vi "HEWH RLT PRAT.vi"() -> ()   [LabVIEW 2023] (continued)
                n1268 = local read "Station B Test Sequence"() -> (w3112:T15[])
                n1269 = local read "Scan Rate (Seconds)"() -> (w3095:T11)
                n1270 = property on="Start/Pause test" class="Bool (strict)"("DisabledEnum"=T87."Enabled" ("Disabled")) -> ()  [unwired: 2 in, 2 out]
                n1271 = Bundle By Name(cluster=T89 {"Test Fixture Hardware"={"Power "={"Yokogawa"={"WT210"={"Sample Rate (1: 0.25s)"=0, "A Range (12: 20A)"=0, "V Range (6: 600V)"=0, "Power VISA Yokogawa WT210"=""}, "WT500"={"Power VISA Yokogawa WT500"="", "V Range (8: 1000V)"=0, "I Range (7: 40A)"=0, "Update Rate (3: 500ms)"=0}, "WT310_2"={"Sample Rate (1: 0.25s)"=0, "A Range (12: 20A)"=0, "V Range (6: 600V)"=0, "Power VISA Yokogawa WT310_2"=""}, "WT310_3"={"Sample Rate (1: 0.25s)"=0, "A Range (12: 20A)"=0, "V Range (6: 600V)"=0, "Power VISA Yokogawa WT310_3"=""}}, "Aplus"={"Aplus IP Address"="", "Remote Port"=0, "Instrument"="", "Instr Driver Revision"=""}, "Power Limits"={"Crest Factor"={"Upper Limit"=0.0, "Lower Limit"=0.0}, "Harmonic Content"={"Uthd"=0.0}, "Voltage"={"% Error"=0.0}, "Stability"={"<1 Watt "={"Wattage"=0.0, "Slope (mW/H)"=0.0}, ">1 Watt"={"1%Power/Hour"=0.0}}}, "Nominal Voltage"=0, "Time Limit (s)"=0.0, "Power Variation Limit (%)"=0.0, "Power Supply"={"Chroma 61605"="", "Use Chroma?"=FALSE}}, "Weight Scale"={"Com Options"={"IND560Scale VISA"="", "IP Address"="", "Remote Port"=0, "Setra Scale VISA"="", "GSE 350"=""}, "Select Scale"=""}, "Flow Rates"={"Laurel Cold IP Address"="", "Laurel Hot IP Address"="", "Hot Water Laurel VISA"="", "Cold Water Laurel VISA"="", "Remote Port"=0, "Laurel Communication Type"="", "Meters To Collect (Hot Cold)"="", "HOT Laurel Reference"=refnum, "COLD Laurel Reference"=refnum, "Modbus Hot Ref"=refnum}, "Analog Data"={"Agilent"={"Agilent 34972_1"="", "Agilent 34972_2"="", "Agilent 34972_3"="", "Agilent 34972_4"="", "Agilent 34972_5"="", "Agilent 34972_6"="", "Agilent Gain"=0.0, "TC Type (K,J,T)"="", "Instrument IDN?"="", "TC Channels-List"="", "Analog Channels-List"="", "Agilent Cluster Array"=[], "TC Channels-List 2"="", "Analog Channels-List 2"=""}, "Yokogawa"={"MW100"="", "Intellifaucet"=FALSE}, "Select Analog"="", "TC Coefficients"={"TC Coefficients 1"=[], "TC Coefficients 2"=[], "TC Coefficients 3"=[], "TC Coefficients 4"=[], "TC Coefficients 5"=[], "TC Coefficients 6"=[], "TC Coefficients 7"=[]}, "NI Tasks (Dryer DOE)"=[], "Laurel Analog"={"Laurel IP (Water Temp)"="", "Laurel IP (Pressure)"=""}}, "Viasala Temperature & Humidity"={"IP Address 1"="", "Remote Port"=0, "IP Address 2"="", "IP Address 3"="", "Viasala Modbus"=refnum, "Probe Number"=0}, "Gas Meter"={"Gas Meter 1"="", "Gas Meter 2"="", "Gas Meter 3"="", "Gas Meter 4"="", "Gas Meter 5"="", "Gas Meter 6"="", "Data Frame Format"={"Absolute Pressure"=FALSE, "Gauge/Diff. Pressure"=FALSE, "Barometric Pressure"=FALSE, "Temperature"=FALSE, "Volumetric"=FALSE, "Mass"=FALSE, "Setpoint"=FALSE, "Valve Drive"=FALSE, "Totalizer"=FALSE, "Totalizer Timer"=FALSE, "Totalizer Average Flow"=FALSE, "Totalizer Peak Flow"=FALSE, "Gas Selected"=FALSE, "Tot. Timer Format"=0}, "Measurement Units"={"Software Rev"="", "Model Number"="", "Manufacturer Info"="", "Software Sub-Rev"="", "Board Rev"="", "Units of Measure Input"={"Abs. Pressure"="", "Gauge/Diff. Press."="", "Barometric Press."="", "Temperature"="", "Volume"="", "Mass"="", "Setpoint"="", "Valve Drive"="", "Totalizer"="", "Tot. Timer"="", "Tot. Avg. Flow"="", "Tot. Peak Flow"=""}}, "Ritter Gas Meter 1"=""}, "Barometric Pressure"={"HEISE 901A"="", "Use Barometer?"=FALSE}, "Gas Analysis"={"Ultramat 23 VISA"=""}, "Inficon Micro GC"={"Propane IP Address"="192.168.1.33", "Natural Gas  IP Address"="192.168.1.32", "Remote Port"=502, "Natural Modbus"=refnum, "Propane Modbus"=refnum}, "Tenney Environmental Chamber"={"Remote Port"=0, "IP Address"="", "Tenney Modbus"=refnum}}, "GEA2"={"Address"=0, "Source"=0, "Viper/Hawk"=0}, "DOE Capacity Measurments"={"Weight 1"=0.0, "Model Number 1"="", "Temp 1"=0.0, "Serial Number 1"="", "Lab Number 1"="", "Lab Number 2"="", "Serial Number 2"="", "Temp 2"=0.0, "Model Number 2"="", "Weight 2"=0.0, "Lab Number 3"="", "Serial Number 3"="", "Temp 3"=0.0, "Model Number 3"="", "Weight 3"=0.0, "Lab Number 4"="", "Serial Number 4"="", "Temp 4"=0.0, "Model Number 4"="", "Weight 4"=0.0, "Capacity Measurment Output String"=[]}, "Initialize.Washer In"={"Appliance Details"={"FileVersionInfo"={"FileVersion"="", "ProductName"="", "InternalName"="", "CompanyName"="", "LegalCopyright"="", "FileDescription"=""}, "Dishwasher Info"={"Open Cup Weight (gm):"=0.0, "Auto Cup Weight (gm):"=0.0, "Detergent-Dish:"="", "Inlet Temperature-Dish:"="", "Cycle Mode-Dish:"="", "Unit Control-Dish:"="", "Manufacturer-Dish:"=""}, "Washer Info"={"Hot Water Temperature (Fahrenheit):"="", "Cold Water Temperature (Fahrenheit):"="", "Capacity (cu.ft):"=0.0, "Initial Cloth Weight:"=0.0, "Cloth Lot:"=0, "Model Family:"="", "Program Name:"="", "Cycle Selection:"="", "Wash Temperature:"="", "Rinse Temperature:"="", "Load Size:"=""}, "File Name Output Array"=[], "Calibration Output Array"=[], "Appliance Common"={"Engineer:"="", "Model Number:"="", "Serial Number:"="", "Comments:"="", "Station ID:"="", "Technician:"="", "TR Number:"="", "Lab ID:"="", "Voltage:"="", "Water Pressure (PSI):"="", "Test Date:"="", "Computer Name:"="", "IP Address:"="", "Ambient RH:"="", "Frequency:"="", "Build:"="", "Filename:"="", "Test Type:"="", "Load Run #:"=0, "Ambient Temperature (F):"="", "File Path:"=path "", "Cycles Per Year"=0}, "Water Heater"={"Heating Mode:"=""}, "Dryer"={"Heat Setting:"="", "Washer Water Temperature (60 ± 5°F):"=0, "Water Hardness (PPM):"=0, "Dryness Setting:"="", "Dryer Type:"="", "Exhaust:"="", "Drying Cycle:"="", "Load Type:"="", "Nominal Load Weight"="", "Dryer Initial IMC Data"={"Measured IMC (lbs)"=0.0, "Actual Initial RMC (%)"=0.0, "RMC (Desired %)"=0.0, "Bone Dry Wt(lbs)"=0.0, "Tolerance(%)"=0.0, "Actual Final RMC (%)"=0.0, "CEF (lbf/kWh)"=0.0, "Minimum Weight (lbf)"=0.0, "Average Weight (lbf)"=0.0, "Maximum Weight (lbf)"=0.0, "Measured IMC In Range?"=FALSE, "Moisture Reduction Factor"=0.0, "Field Use Factor"=0.0, "Empty Dryer Cold Weigth"=0.0, "Energy Standard"=enum."D2-Automatic Dryer", "Weight Cloth (lbs)"=0.0, "Relative Moisture Content (%)"=0.0, "Relative Moisture Content - Avg (%)"=0.0}}}, "Display Data (RLT)"={"Status Color"=0, "Serial Number Display"="", "Cycle Count Display"=0, "Station Label Display"="", "Current Run Start Time Display"=0.0, "Board ID Display"="", "RPM Display"=0, "Current Display"=0.0, "Current Path Display"=path "", "Saving Display"=FALSE, "Unit Type Display"=enum."", "Total Time On Display"=0.0, "UI Button"=FALSE}}} ("Washer Controls In"), "Initialize.Washer In.Display Data (RLT).Station Label Display"=w3100) -> (w3099:T89)
                n1272 = local read "File Locations B"() -> (w3108:T3)
                n1273 = Unbundle By Name(w3110) -> ("LV Program"=w3109:T25)
                n1274 = call "PRAT Test Setup.vi"("Station Input"="B", "Test Sequence Input"=w3112, "Input Scan Rate"=w3095, "Washer Controls In"=w3099, "Filepath In"=w3108, "Error In"=w3122, "LV Program"=w3109) -> ("Cutout Delay (sec)"=w3104:dbl, "NOx Purge Time Out"=w3091:dbl, "Disable Purge Pressurization Output"=w3096:bool, "Unit Setpoint Out"=w3102:i32, "Appliance Details"=w3106:T5, "Filepath Out"=w3107:T3, "Station ID"=w3118:T26, "Log Data Output"=w3105:bool, "Temperature Decline Amount (°F)"=w3093:dbl, "Final Output"=w3121:T15[], "PRAT Test.ctlCancel Output"=w3119:bool, "Scan Rate Output"=w3094:dbl, "Test Procedure"=w3097:string, "Reset Cycle Count"=w3114:bool, "New Cycle Count Out"=→"Updated Cycle Count":i32, "Purge Time (s)"=w3092:dbl, "Error Out"=w3117:errorcluster)  [unwired: 4 in]
                n1275 = local write "Reset Cycle Count"(w3114) -> ()
                n1276 = case shown="False" w3119 {
                  tunnel: w3121 -> [w3145 _]
                  tunnel: w3118 -> [w3144 _]
                  tunnel: w3117 -> [w3141 w3147]
                  tunnel: [w3138 w3147] -> w3116
                  tunnel: w3115 -> [w3143 _]
                  tunnel: w3111 -> [w3137 _]
                  tunnel: w3107 -> [w3135 _]
                  tunnel: w3106 -> [w3136 _]
                  tunnel: w3105 -> [w3134 _]
                  tunnel: w3104 -> [w3133 _]
                  tunnel: w3102 -> [w3131 _]
                  tunnel: w3097 -> [w3130 _]
                  tunnel: w3096 -> [w3126 _]
                  tunnel: w3094 -> [w3125 _]
                  tunnel: w3093 -> [w3129 _]
                  tunnel: w3092 -> [w3128 _]
                  tunnel: w3091 -> [w3127 _]
                  frame False {
                    n1277 = local write "Station ID to Reset"(w3144) -> ()
                    n1278 = local write "StationB Setpoint"(w3131) -> ()
                    n1279 = local write "Temperature Decline Amount (°F)"(w3129) -> ()
                    n1280 = Generate User Event(user event=w3143, event data cluster=TRUE ("event data"), error in=w3141) -> (error out=w3139:errorcluster)  [unwired: 1 in, 1 out]
                    n1281 = local write "Cutout Delay B (sec)"(w3133) -> ()
                    n1282 = local write "Purge Time (Seconds)"(w3128) -> ()
                    n1283 = local write "NOx Purge Time"(w3127) -> ()
                    n1284 = local write "Disable Station 2"(HEWH_RLT_Station_Disable."Enable Station" ("Disable Station 2")) -> ()
                    n1285 = Generate User Event(user event=w3137, event data cluster=TRUE ("event data"), error in=w3139) -> (error out=w3138:errorcluster)  [unwired: 1 in, 1 out]
                    n1286 = case shown="True" w3126 {
                      frame False {
                      }
                      frame True {
                        n1287 = local write "Pressurization Time (sec)"(0 ("Pressurization Time (sec)")) -> ()
                      }
                    }
                    n1288 = property on="Scan Rate (Seconds)" class="DigNum (strict)"("Value"=w3125) -> ()  [unwired: 2 in, 2 out]
                    "Station B Test Sequence" <- w3145
                    "Appliance Details B" <- w3136
                    "Updated File Path B" <- w3135
                    "Log Data Output (B)" <- w3134
                    "Test Procedure 2" <- w3130
                    "Disable Purge Pressurization B" <- w3126
                  }
                  frame True {
                  }
                }
              }
              event Value Change {
                n1289 = event-data() -> ()  [unwired: 1 in, 6 out]
                n1290 = Unbundle By Name(w3156) -> ("Display Data (RLT).Station Label Display"=w3157:string)
                n1291 = local read "Core HEWH Data Input C"() -> (w3167:T13)
                n1292 = local read "Station C Test Sequence"() -> (w3169:T15[])
                n1293 = local read "Scan Rate (Seconds)"() -> (w3151:T11)
                n1294 = property on="Start/Pause test" class="Bool (strict)"("DisabledEnum"=T87."Enabled" ("Disabled")) -> ()  [unwired: 2 in, 2 out]
                n1295 = Bundle By Name(cluster=T89 {"Test Fixture Hardware"={"Power "={"Yokogawa"={"WT210"={"Sample Rate (1: 0.25s)"=0, "A Range (12: 20A)"=0, "V Range (6: 600V)"=0, "Power VISA Yokogawa WT210"=""}, "WT500"={"Power VISA Yokogawa WT500"="", "V Range (8: 1000V)"=0, "I Range (7: 40A)"=0, "Update Rate (3: 500ms)"=0}, "WT310_2"={"Sample Rate (1: 0.25s)"=0, "A Range (12: 20A)"=0, "V Range (6: 600V)"=0, "Power VISA Yokogawa WT310_2"=""}, "WT310_3"={"Sample Rate (1: 0.25s)"=0, "A Range (12: 20A)"=0, "V Range (6: 600V)"=0, "Power VISA Yokogawa WT310_3"=""}}, "Aplus"={"Aplus IP Address"="", "Remote Port"=0, "Instrument"="", "Instr Driver Revision"=""}, "Power Limits"={"Crest Factor"={"Upper Limit"=0.0, "Lower Limit"=0.0}, "Harmonic Content"={"Uthd"=0.0}, "Voltage"={"% Error"=0.0}, "Stability"={"<1 Watt "={"Wattage"=0.0, "Slope (mW/H)"=0.0}, ">1 Watt"={"1%Power/Hour"=0.0}}}, "Nominal Voltage"=0, "Time Limit (s)"=0.0, "Power Variation Limit (%)"=0.0, "Power Supply"={"Chroma 61605"="", "Use Chroma?"=FALSE}}, "Weight Scale"={"Com Options"={"IND560Scale VISA"="", "IP Address"="", "Remote Port"=0, "Setra Scale VISA"="", "GSE 350"=""}, "Select Scale"=""}, "Flow Rates"={"Laurel Cold IP Address"="", "Laurel Hot IP Address"="", "Hot Water Laurel VISA"="", "Cold Water Laurel VISA"="", "Remote Port"=0, "Laurel Communication Type"="", "Meters To Collect (Hot Cold)"="", "HOT Laurel Reference"=refnum, "COLD Laurel Reference"=refnum, "Modbus Hot Ref"=refnum}, "Analog Data"={"Agilent"={"Agilent 34972_1"="", "Agilent 34972_2"="", "Agilent 34972_3"="", "Agilent 34972_4"="", "Agilent 34972_5"="", "Agilent 34972_6"="", "Agilent Gain"=0.0, "TC Type (K,J,T)"="", "Instrument IDN?"="", "TC Channels-List"="", "Analog Channels-List"="", "Agilent Cluster Array"=[], "TC Channels-List 2"="", "Analog Channels-List 2"=""}, "Yokogawa"={"MW100"="", "Intellifaucet"=FALSE}, "Select Analog"="", "TC Coefficients"={"TC Coefficients 1"=[], "TC Coefficients 2"=[], "TC Coefficients 3"=[], "TC Coefficients 4"=[], "TC Coefficients 5"=[], "TC Coefficients 6"=[], "TC Coefficients 7"=[]}, "NI Tasks (Dryer DOE)"=[], "Laurel Analog"={"Laurel IP (Water Temp)"="", "Laurel IP (Pressure)"=""}}, "Viasala Temperature & Humidity"={"IP Address 1"="", "Remote Port"=0, "IP Address 2"="", "IP Address 3"="", "Viasala Modbus"=refnum, "Probe Number"=0}, "Gas Meter"={"Gas Meter 1"="", "Gas Meter 2"="", "Gas Meter 3"="", "Gas Meter 4"="", "Gas Meter 5"="", "Gas Meter 6"="", "Data Frame Format"={"Absolute Pressure"=FALSE, "Gauge/Diff. Pressure"=FALSE, "Barometric Pressure"=FALSE, "Temperature"=FALSE, "Volumetric"=FALSE, "Mass"=FALSE, "Setpoint"=FALSE, "Valve Drive"=FALSE, "Totalizer"=FALSE, "Totalizer Timer"=FALSE, "Totalizer Average Flow"=FALSE, "Totalizer Peak Flow"=FALSE, "Gas Selected"=FALSE, "Tot. Timer Format"=0}, "Measurement Units"={"Software Rev"="", "Model Number"="", "Manufacturer Info"="", "Software Sub-Rev"="", "Board Rev"="", "Units of Measure Input"={"Abs. Pressure"="", "Gauge/Diff. Press."="", "Barometric Press."="", "Temperature"="", "Volume"="", "Mass"="", "Setpoint"="", "Valve Drive"="", "Totalizer"="", "Tot. Timer"="", "Tot. Avg. Flow"="", "Tot. Peak Flow"=""}}, "Ritter Gas Meter 1"=""}, "Barometric Pressure"={"HEISE 901A"="", "Use Barometer?"=FALSE}, "Gas Analysis"={"Ultramat 23 VISA"=""}, "Inficon Micro GC"={"Propane IP Address"="192.168.1.33", "Natural Gas  IP Address"="192.168.1.32", "Remote Port"=502, "Natural Modbus"=refnum, "Propane Modbus"=refnum}, "Tenney Environmental Chamber"={"Remote Port"=0, "IP Address"="", "Tenney Modbus"=refnum}}, "GEA2"={"Address"=0, "Source"=0, "Viper/Hawk"=0}, "DOE Capacity Measurments"={"Weight 1"=0.0, "Model Number 1"="", "Temp 1"=0.0, "Serial Number 1"="", "Lab Number 1"="", "Lab Number 2"="", "Serial Number 2"="", "Temp 2"=0.0, "Model Number 2"="", "Weight 2"=0.0, "Lab Number 3"="", "Serial Number 3"="", "Temp 3"=0.0, "Model Number 3"="", "Weight 3"=0.0, "Lab Number 4"="", "Serial Number 4"="", "Temp 4"=0.0, "Model Number 4"="", "Weight 4"=0.0, "Capacity Measurment Output String"=[]}, "Initialize.Washer In"={"Appliance Details"={"FileVersionInfo"={"FileVersion"="", "ProductName"="", "InternalName"="", "CompanyName"="", "LegalCopyright"="", "FileDescription"=""}, "Dishwasher Info"={"Open Cup Weight (gm):"=0.0, "Auto Cup Weight (gm):"=0.0, "Detergent-Dish:"="", "Inlet Temperature-Dish:"="", "Cycle Mode-Dish:"="", "Unit Control-Dish:"="", "Manufacturer-Dish:"=""}, "Washer Info"={"Hot Water Temperature (Fahrenheit):"="", "Cold Water Temperature (Fahrenheit):"="", "Capacity (cu.ft):"=0.0, "Initial Cloth Weight:"=0.0, "Cloth Lot:"=0, "Model Family:"="", "Program Name:"="", "Cycle Selection:"="", "Wash Temperature:"="", "Rinse Temperature:"="", "Load Size:"=""}, "File Name Output Array"=[], "Calibration Output Array"=[], "Appliance Common"={"Engineer:"="", "Model Number:"="", "Serial Number:"="", "Comments:"="", "Station ID:"="", "Technician:"="", "TR Number:"="", "Lab ID:"="", "Voltage:"="", "Water Pressure (PSI):"="", "Test Date:"="", "Computer Name:"="", "IP Address:"="", "Ambient RH:"="", "Frequency:"="", "Build:"="", "Filename:"="", "Test Type:"="", "Load Run #:"=0, "Ambient Temperature (F):"="", "File Path:"=path "", "Cycles Per Year"=0}, "Water Heater"={"Heating Mode:"=""}, "Dryer"={"Heat Setting:"="", "Washer Water Temperature (60 ± 5°F):"=0, "Water Hardness (PPM):"=0, "Dryness Setting:"="", "Dryer Type:"="", "Exhaust:"="", "Drying Cycle:"="", "Load Type:"="", "Nominal Load Weight"="", "Dryer Initial IMC Data"={"Measured IMC (lbs)"=0.0, "Actual Initial RMC (%)"=0.0, "RMC (Desired %)"=0.0, "Bone Dry Wt(lbs)"=0.0, "Tolerance(%)"=0.0, "Actual Final RMC (%)"=0.0, "CEF (lbf/kWh)"=0.0, "Minimum Weight (lbf)"=0.0, "Average Weight (lbf)"=0.0, "Maximum Weight (lbf)"=0.0, "Measured IMC In Range?"=FALSE, "Moisture Reduction Factor"=0.0, "Field Use Factor"=0.0, "Empty Dryer Cold Weigth"=0.0, "Energy Standard"=enum."D2-Automatic Dryer", "Weight Cloth (lbs)"=0.0, "Relative Moisture Content (%)"=0.0, "Relative Moisture Content - Avg (%)"=0.0}}}, "Display Data (RLT)"={"Status Color"=0, "Serial Number Display"="", "Cycle Count Display"=0, "Station Label Display"="", "Current Run Start Time Display"=0.0, "Board ID Display"="", "RPM Display"=0, "Current Display"=0.0, "Current Path Display"=path "", "Saving Display"=FALSE, "Unit Type Display"=enum."", "Total Time On Display"=0.0, "UI Button"=FALSE}}} ("Washer Controls In"), "Initialize.Washer In.Display Data (RLT).Station Label Display"=w3157) -> (w3155:T89)
                n1296 = local read "File Locations C"() -> (w3165:T3)
                n1297 = Unbundle By Name(w3167) -> ("LV Program"=w3166:T25)
                n1298 = call "PRAT Test Setup.vi"("Station Input"="C", "Test Sequence Input"=w3169, "Input Scan Rate"=w3151, "Washer Controls In"=w3155, "Filepath In"=w3165, "Error In"=w3179, "LV Program"=w3166) -> ("Cutout Delay (sec)"=w3161:dbl, "NOx Purge Time Out"=w3148:dbl, "Disable Purge Pressurization Output"=w3153:bool, "Unit Setpoint Out"=w3159:i32, "Appliance Details"=w3163:T5, "Filepath Out"=w3164:T3, "Station ID"=w3176:T26, "Log Data Output"=w3162:bool, "Temperature Decline Amount (°F)"=w3150:dbl, "Final Output"=w3178:T15[], "PRAT Test.ctlCancel Output"=w3172:bool, "Scan Rate Output"=w3152:dbl, "Test Procedure"=w3154:string, "Reset Cycle Count"=→"Reset Cycle Count":bool, "New Cycle Count Out"=w3170:i32, "Purge Time (s)"=w3149:dbl, "Error Out"=w3175:errorcluster)  [unwired: 4 in]
                n1299 = local write "Updated Cycle Count"(w3170) -> ()
                n1300 = case shown="False" w3172 {
                  tunnel: w3178 -> [w3202 _]
                  tunnel: w3176 -> [w3201 _]
                  tunnel: w3175 -> [w3198 w3204]
                  tunnel: [w3195 w3204] -> w3174
                  tunnel: w3173 -> [w3199 _]
                  tunnel: w3168 -> [w3194 _]
                  tunnel: w3164 -> [w3192 _]
                  tunnel: w3163 -> [w3193 _]
                  tunnel: w3162 -> [w3191 _]
                  tunnel: w3161 -> [w3190 _]
                  tunnel: w3159 -> [w3188 _]
                  tunnel: w3154 -> [w3187 _]
                  tunnel: w3153 -> [w3183 _]
                  tunnel: w3152 -> [w3182 _]
                  tunnel: w3150 -> [w3186 _]
                  tunnel: w3149 -> [w3185 _]
                  tunnel: w3148 -> [w3184 _]
                  frame False {
                    n1301 = local write "Station ID to Reset"(w3201) -> ()
                    n1302 = local write "Purge Time (Seconds)"(w3185) -> ()
                    n1303 = local write "Temperature Decline Amount (°F)"(w3186) -> ()
                    n1304 = local write "StationC Setpoint"(w3188) -> ()
                    n1305 = Generate User Event(user event=w3199, event data cluster=TRUE ("event data"), error in=w3198) -> (error out=w3196:errorcluster)  [unwired: 1 in, 1 out]
                    n1306 = local write "Disable Station 3"(HEWH_RLT_Station_Disable."Enable Station" ("Disable Station 3")) -> ()
                    n1307 = local write "Cutout Delay C (sec)"(w3190) -> ()
                    n1308 = local write "NOx Purge Time"(w3184) -> ()
                    n1309 = case shown="True" w3183 {
                      frame False {
                      }
                      frame True {
                        n1310 = local write "Pressurization Time (sec)"(0 ("Pressurization Time (sec)")) -> ()
                      }
                    }
                    n1311 = Generate User Event(user event=w3194, event data cluster=TRUE ("event data"), error in=w3196) -> (error out=w3195:errorcluster)  [unwired: 1 in, 1 out]
                    n1312 = property on="Scan Rate (Seconds)" class="DigNum (strict)"("Value"=w3182) -> ()  [unwired: 2 in, 2 out]
                    "Station C Test Sequence" <- w3202
                    "Appliance Details C" <- w3193
                    "Updated File Path C" <- w3192
                    "Log Data Output (C)" <- w3191
                    "Test Procedure 3" <- w3187
                    "Disable Purge Pressurization C" <- w3183
                  }
                  frame True {
                  }
                }
              }
              event Value Change {
                n1313 = event-data() -> ()  [unwired: 1 in, 6 out]
                n1314 = Unbundle By Name(w3213) -> ("Display Data (RLT).Station Label Display"=w3214:string)
                n1315 = local read "Core HEWH Data Input D"() -> (w3224:T13)
                n1316 = local read "Station D Test Sequence"() -> (w3226:T15[])
                n1317 = local read "Scan Rate (Seconds)"() -> (w3208:T11)
                n1318 = Bundle By Name(cluster=T89 {"Test Fixture Hardware"={"Power "={"Yokogawa"={"WT210"={"Sample Rate (1: 0.25s)"=0, "A Range (12: 20A)"=0, "V Range (6: 600V)"=0, "Power VISA Yokogawa WT210"=""}, "WT500"={"Power VISA Yokogawa WT500"="", "V Range (8: 1000V)"=0, "I Range (7: 40A)"=0, "Update Rate (3: 500ms)"=0}, "WT310_2"={"Sample Rate (1: 0.25s)"=0, "A Range (12: 20A)"=0, "V Range (6: 600V)"=0, "Power VISA Yokogawa WT310_2"=""}, "WT310_3"={"Sample Rate (1: 0.25s)"=0, "A Range (12: 20A)"=0, "V Range (6: 600V)"=0, "Power VISA Yokogawa WT310_3"=""}}, "Aplus"={"Aplus IP Address"="", "Remote Port"=0, "Instrument"="", "Instr Driver Revision"=""}, "Power Limits"={"Crest Factor"={"Upper Limit"=0.0, "Lower Limit"=0.0}, "Harmonic Content"={"Uthd"=0.0}, "Voltage"={"% Error"=0.0}, "Stability"={"<1 Watt "={"Wattage"=0.0, "Slope (mW/H)"=0.0}, ">1 Watt"={"1%Power/Hour"=0.0}}}, "Nominal Voltage"=0, "Time Limit (s)"=0.0, "Power Variation Limit (%)"=0.0, "Power Supply"={"Chroma 61605"="", "Use Chroma?"=FALSE}}, "Weight Scale"={"Com Options"={"IND560Scale VISA"="", "IP Address"="", "Remote Port"=0, "Setra Scale VISA"="", "GSE 350"=""}, "Select Scale"=""}, "Flow Rates"={"Laurel Cold IP Address"="", "Laurel Hot IP Address"="", "Hot Water Laurel VISA"="", "Cold Water Laurel VISA"="", "Remote Port"=0, "Laurel Communication Type"="", "Meters To Collect (Hot Cold)"="", "HOT Laurel Reference"=refnum, "COLD Laurel Reference"=refnum, "Modbus Hot Ref"=refnum}, "Analog Data"={"Agilent"={"Agilent 34972_1"="", "Agilent 34972_2"="", "Agilent 34972_3"="", "Agilent 34972_4"="", "Agilent 34972_5"="", "Agilent 34972_6"="", "Agilent Gain"=0.0, "TC Type (K,J,T)"="", "Instrument IDN?"="", "TC Channels-List"="", "Analog Channels-List"="", "Agilent Cluster Array"=[], "TC Channels-List 2"="", "Analog Channels-List 2"=""}, "Yokogawa"={"MW100"="", "Intellifaucet"=FALSE}, "Select Analog"="", "TC Coefficients"={"TC Coefficients 1"=[], "TC Coefficients 2"=[], "TC Coefficients 3"=[], "TC Coefficients 4"=[], "TC Coefficients 5"=[], "TC Coefficients 6"=[], "TC Coefficients 7"=[]}, "NI Tasks (Dryer DOE)"=[], "Laurel Analog"={"Laurel IP (Water Temp)"="", "Laurel IP (Pressure)"=""}}, "Viasala Temperature & Humidity"={"IP Address 1"="", "Remote Port"=0, "IP Address 2"="", "IP Address 3"="", "Viasala Modbus"=refnum, "Probe Number"=0}, "Gas Meter"={"Gas Meter 1"="", "Gas Meter 2"="", "Gas Meter 3"="", "Gas Meter 4"="", "Gas Meter 5"="", "Gas Meter 6"="", "Data Frame Format"={"Absolute Pressure"=FALSE, "Gauge/Diff. Pressure"=FALSE, "Barometric Pressure"=FALSE, "Temperature"=FALSE, "Volumetric"=FALSE, "Mass"=FALSE, "Setpoint"=FALSE, "Valve Drive"=FALSE, "Totalizer"=FALSE, "Totalizer Timer"=FALSE, "Totalizer Average Flow"=FALSE, "Totalizer Peak Flow"=FALSE, "Gas Selected"=FALSE, "Tot. Timer Format"=0}, "Measurement Units"={"Software Rev"="", "Model Number"="", "Manufacturer Info"="", "Software Sub-Rev"="", "Board Rev"="", "Units of Measure Input"={"Abs. Pressure"="", "Gauge/Diff. Press."="", "Barometric Press."="", "Temperature"="", "Volume"="", "Mass"="", "Setpoint"="", "Valve Drive"="", "Totalizer"="", "Tot. Timer"="", "Tot. Avg. Flow"="", "Tot. Peak Flow"=""}}, "Ritter Gas Meter 1"=""}, "Barometric Pressure"={"HEISE 901A"="", "Use Barometer?"=FALSE}, "Gas Analysis"={"Ultramat 23 VISA"=""}, "Inficon Micro GC"={"Propane IP Address"="192.168.1.33", "Natural Gas  IP Address"="192.168.1.32", "Remote Port"=502, "Natural Modbus"=refnum, "Propane Modbus"=refnum}, "Tenney Environmental Chamber"={"Remote Port"=0, "IP Address"="", "Tenney Modbus"=refnum}}, "GEA2"={"Address"=0, "Source"=0, "Viper/Hawk"=0}, "DOE Capacity Measurments"={"Weight 1"=0.0, "Model Number 1"="", "Temp 1"=0.0, "Serial Number 1"="", "Lab Number 1"="", "Lab Number 2"="", "Serial Number 2"="", "Temp 2"=0.0, "Model Number 2"="", "Weight 2"=0.0, "Lab Number 3"="", "Serial Number 3"="", "Temp 3"=0.0, "Model Number 3"="", "Weight 3"=0.0, "Lab Number 4"="", "Serial Number 4"="", "Temp 4"=0.0, "Model Number 4"="", "Weight 4"=0.0, "Capacity Measurment Output String"=[]}, "Initialize.Washer In"={"Appliance Details"={"FileVersionInfo"={"FileVersion"="", "ProductName"="", "InternalName"="", "CompanyName"="", "LegalCopyright"="", "FileDescription"=""}, "Dishwasher Info"={"Open Cup Weight (gm):"=0.0, "Auto Cup Weight (gm):"=0.0, "Detergent-Dish:"="", "Inlet Temperature-Dish:"="", "Cycle Mode-Dish:"="", "Unit Control-Dish:"="", "Manufacturer-Dish:"=""}, "Washer Info"={"Hot Water Temperature (Fahrenheit):"="", "Cold Water Temperature (Fahrenheit):"="", "Capacity (cu.ft):"=0.0, "Initial Cloth Weight:"=0.0, "Cloth Lot:"=0, "Model Family:"="", "Program Name:"="", "Cycle Selection:"="", "Wash Temperature:"="", "Rinse Temperature:"="", "Load Size:"=""}, "File Name Output Array"=[], "Calibration Output Array"=[], "Appliance Common"={"Engineer:"="", "Model Number:"="", "Serial Number:"="", "Comments:"="", "Station ID:"="", "Technician:"="", "TR Number:"="", "Lab ID:"="", "Voltage:"="", "Water Pressure (PSI):"="", "Test Date:"="", "Computer Name:"="", "IP Address:"="", "Ambient RH:"="", "Frequency:"="", "Build:"="", "Filename:"="", "Test Type:"="", "Load Run #:"=0, "Ambient Temperature (F):"="", "File Path:"=path "", "Cycles Per Year"=0}, "Water Heater"={"Heating Mode:"=""}, "Dryer"={"Heat Setting:"="", "Washer Water Temperature (60 ± 5°F):"=0, "Water Hardness (PPM):"=0, "Dryness Setting:"="", "Dryer Type:"="", "Exhaust:"="", "Drying Cycle:"="", "Load Type:"="", "Nominal Load Weight"="", "Dryer Initial IMC Data"={"Measured IMC (lbs)"=0.0, "Actual Initial RMC (%)"=0.0, "RMC (Desired %)"=0.0, "Bone Dry Wt(lbs)"=0.0, "Tolerance(%)"=0.0, "Actual Final RMC (%)"=0.0, "CEF (lbf/kWh)"=0.0, "Minimum Weight (lbf)"=0.0, "Average Weight (lbf)"=0.0, "Maximum Weight (lbf)"=0.0, "Measured IMC In Range?"=FALSE, "Moisture Reduction Factor"=0.0, "Field Use Factor"=0.0, "Empty Dryer Cold Weigth"=0.0, "Energy Standard"=enum."D2-Automatic Dryer", "Weight Cloth (lbs)"=0.0, "Relative Moisture Content (%)"=0.0, "Relative Moisture Content - Avg (%)"=0.0}}}, "Display Data (RLT)"={"Status Color"=0, "Serial Number Display"="", "Cycle Count Display"=0, "Station Label Display"="", "Current Run Start Time Display"=0.0, "Board ID Display"="", "RPM Display"=0, "Current Display"=0.0, "Current Path Display"=path "", "Saving Display"=FALSE, "Unit Type Display"=enum."", "Total Time On Display"=0.0, "UI Button"=FALSE}}} ("Washer Controls In"), "Initialize.Washer In.Display Data (RLT).Station Label Display"=w3214) -> (w3212:T89)
                n1319 = local read "File Locations D"() -> (w3220:T3)
                n1320 = property on="Start/Pause test" class="Bool (strict)"("DisabledEnum"=T87."Enabled" ("Disabled")) -> ()  [unwired: 2 in, 2 out]
                n1321 = Unbundle By Name(w3224) -> ("LV Program"=w3223:T25)
                n1322 = call "PRAT Test Setup.vi"("Station Input"="D", "Test Sequence Input"=w3226, "Input Scan Rate"=w3208, "Washer Controls In"=w3212, "Filepath In"=w3220, "Error In"=w3236, "LV Program"=w3223) -> ("Cutout Delay (sec)"=w3218:dbl, "NOx Purge Time Out"=w3205:dbl, "Disable Purge Pressurization Output"=w3210:bool, "Unit Setpoint Out"=w3216:i32, "Appliance Details"=w3221:T5, "Filepath Out"=w3222:T3, "Station ID"=w3230:T26, "Log Data Output"=w3219:bool, "Temperature Decline Amount (°F)"=w3207:dbl, "Final Output"=w3235:T15[], "PRAT Test.ctlCancel Output"=w3233:bool, "Scan Rate Output"=w3209:dbl, "Test Procedure"=w3211:string, "Reset Cycle Count"=w3228:bool, "New Cycle Count Out"=w3227:i32, "Purge Time (s)"=w3206:dbl, "Error Out"=w3232:errorcluster)  [unwired: 4 in]
                n1323 = local write "Updated Cycle Count"(w3227) -> ()
                n1324 = local write "Reset Cycle Count"(w3228) -> ()
                n1325 = case shown="False" w3233 {
                  tunnel: w3235 -> [w3259 _]
                  tunnel: w3232 -> [w3255 w3261]
                  tunnel: [w3252 w3261] -> w3231
                  tunnel: w3230 -> [w3258 _]
                  tunnel: w3229 -> [w3256 _]
                  tunnel: w3225 -> [w3251 _]
                  tunnel: w3222 -> [w3249 _]
                  tunnel: w3221 -> [w3250 _]
                  tunnel: w3219 -> [w3248 _]
                  tunnel: w3218 -> [w3247 _]
                  tunnel: w3216 -> [w3245 _]
                  tunnel: w3211 -> [w3244 _]
                  tunnel: w3210 -> [w3241 _]
                  tunnel: w3209 -> [w3240 _]
                  tunnel: w3207 -> [w3243 _]
                  tunnel: w3206 -> [w3239 _]
                  tunnel: w3205 -> [w3242 _]
                  frame False {
                    n1326 = local write "Purge Time (Seconds)"(w3239) -> ()
                    n1327 = local write "Temperature Decline Amount (°F)"(w3243) -> ()
                    n1328 = Generate User Event(user event=w3256, event data cluster=TRUE ("event data"), error in=w3255) -> (error out=w3253:errorcluster)  [unwired: 1 in, 1 out]
                    n1329 = local write "StationD Setpoint"(w3245) -> ()
                    n1330 = local write "Disable Station 4"(HEWH_RLT_Station_Disable."Enable Station" ("Disable Station 4")) -> ()
                    n1331 = local write "Cutout Delay D (sec)"(w3247) -> ()
                    n1332 = local write "NOx Purge Time"(w3242) -> ()
                    n1333 = case shown="True" w3241 {
                      frame False {
                      }
                      frame True {
                        n1334 = local write "Pressurization Time (sec)"(0 ("Pressurization Time (sec)")) -> ()
                      }
                    }
                    n1335 = Generate User Event(user event=w3251, event data cluster=TRUE ("event data"), error in=w3253) -> (error out=w3252:errorcluster)  [unwired: 1 in, 1 out]
                    n1336 = property on="Scan Rate (Seconds)" class="DigNum (strict)"("Value"=w3240) -> ()  [unwired: 2 in, 2 out]
                    "Station D Test Sequence" <- w3259
                    "Station ID to Reset" <- w3258
                    "Appliance Details D" <- w3250
                    "Updated File Path D" <- w3249
                    "Log Data Output (D)" <- w3248
                    "Test Procedure 4" <- w3244
                    "Disable Purge Pressurization D" <- w3241
                  }
                  frame True {
                  }
                }
              }
              event Panel Close? {
                n1337 = event-data() -> ()  [unwired: 1 in, 1 out]
                n1338 = call <vilib>:"Add State(s) to Queue__jki_lib_state_machine.vi"("State(s) in Front (\"\")"="Start Shutdown\nExit", "State(s) in (\"\")"=w3267) -> ("States Out"=w3266:string)  [unwired: 13 in]
                n1339 = event-data("Discard?"=TRUE) -> ()  [unwired: 1 in, 1 out]
              }
              event "Start ANSI UI": Value Change {
                n1340 = event-data() -> ("NewVal"=w3273:bool)  [unwired: 1 in, 5 out]
                n1341 = case shown="True" w3273 {
                  tunnel: w3272 -> [w3275 w3278]
                  tunnel: [w3275 w3277] -> w3271
                  frame False {
                  }
                  frame True {
                    n1342 = local read "Software Elapsed Time"() -> (w3276:T29)
                    n1343 = Bundle By Name(cluster=w3278, "Core HEWH Data Input A.ANSI Rate.ANSI Start Time"=w3276) -> (w3277:T103)
                  }
                }
                n1344 = call <vilib>:"Add State(s) to Queue__jki_lib_state_machine.vi"("State(s) in Front (\"\")"="Get Rates" ("State(s) in Front (\"\")"), "State(s) in (\"\")"=w3270) -> ("States Out"=w3269:string)  [unwired: 13 in]
              }
            }
          }
          frame "---------- Core ----------" {
            n1345 = call <vilib>:"Add State(s) to Queue__jki_lib_state_machine.vi"("State(s) in (\"\")"=w3282) -> ("States Out"=w3281:string)  [unwired: 14 in]
          }
          frame Default {
